vi "MecaDrivePoseEst2_New.vi"(4 "VisionMeasurementStdDevs":T4=[[0.9], [0.9], [0.9]], 6 "StateStdDevs":T4=[[0.1], [0.1], [0.1]], 7 "MECA_DRIVE_KINEMATICS":T2={"FrontLeft"={"X"=0.0, "Y"=0.0}, "FrontRight"={"X"=0.0, "Y"=0.0}, "RearLeft"={"X"=0.0, "Y"=0.0}, "RearRight"={"X"=0.0, "Y"=0.0}, "InverseKinematics"=[[0.0, 1.0, -1.0, 0.0], [0.0, 1.0, 1.0, 0.0], [0.0, 1.0, 1.0, 0.0], [0.0, 1.0, -1.0, 0.0]], "ForwardKinematics"=[[0.0, 1.0, -1.0, 0.0], [0.0, 1.0, 1.0, 0.0], [0.0, 1.0, 1.0, 0.0], [0.0, 1.0, -1.0, 0.0]], "PrevCoR"={"X"=0.0, "Y"=0.0}} {"PrevCoR"."Y" format="%14.3f"; "PrevCoR"."X" format="%14.3f"; "RearRight"."Y" format="%14.3f"; "RearRight"."X" format="%14.3f"; "RearLeft"."Y" format="%14.3f"; "RearLeft"."X" format="%14.3f"; "FrontRight"."Y" format="%14.3f"; "FrontRight"."X" format="%14.3f"; "FrontLeft"."Y" format="%14.3f"; "FrontLeft"."X" format="%14.3f"}, 8 "InitialPose":T5={"TRANSLATION"={"X"=0.0, "Y"=0.0}, "ROTATION"={"VALUE"=0.0, "COS"=1.0, "SIN"=0.0}} {"ROTATION"."SIN" format="%13.4f"; "ROTATION"."COS" format="%13.4f"; "ROTATION"."VALUE" format="%13.4f"; "TRANSLATION"."Y" format="%14.3f"; "TRANSLATION"."X" format="%14.3f"}, 10 "Module Positions":T1 {"RearRight" format="%19.3f"; "RearLeft" format="%19.3f"; "FrontRight" format="%19.3f"; "FrontLeft" format="%19.3f"}, 11 "gyroAngle":T6={"VALUE"=0.0, "COS"=1.0, "SIN"=0.0} {"SIN" format="%13.4f"; "COS" format="%13.4f"; "VALUE" format="%13.4f"}) -> (0 "Error":errorcluster, 3 "MecaDrivePoseEstimate":T7={"M_Vision_K"=[], "m_nominal_dT"=0.0, "m_PrevTime_Sec"=0.0, "Pose_Buffer"={"TimeStamps"=[], "DataArray"=[], "Min_TimeStamp"=0.0, "Max_TimeStamp"=0.0, "ItemCount"=0, "MaxBufferTime"=0.0}, "Meca_Drive_Odom"={"POSE"={"TRANSLATION"={"X"=0.0, "Y"=0.0}, "ROTATION"={"VALUE"=0.0, "COS"=1.0, "SIN"=0.0}}, "GyroOffset"={"VALUE"=0.0, "COS"=1.0, "SIN"=0.0}, "PreviousAngle"={"VALUE"=0.0, "COS"=1.0, "SIN"=0.0}, "Kinematics"={"FrontLeft"={"X"=0.0, "Y"=0.0}, "FrontRight"={"X"=0.0, "Y"=0.0}, "RearLeft"={"X"=0.0, "Y"=0.0}, "RearRight"={"X"=0.0, "Y"=0.0}, "InverseKinematics"=[[0.0, 1.0, -1.0, 0.0], [0.0, 1.0, 1.0, 0.0], [0.0, 1.0, 1.0, 0.0], [0.0, 1.0, -1.0, 0.0]], "ForwardKinematics"=[[0.0, 1.0, -1.0, 0.0], [0.0, 1.0, 1.0, 0.0], [0.0, 1.0, 1.0, 0.0], [0.0, 1.0, -1.0, 0.0]], "PrevCoR"={"X"=0.0, "Y"=0.0}}, "PreviousWheelPositions"={"FrontLeft"=0.0, "FrontRight"=0.0, "RearLeft"=0.0, "RearRight"=0.0, "P"=FALSE}}, "M_Q"=[[0.0], [0.0], [0.0]]} {"Meca_Drive_Odom"."PreviousWheelPositions"."RearRight" format="%19.3f"; "Meca_Drive_Odom"."PreviousWheelPositions"."RearLeft" format="%19.3f"; "Meca_Drive_Odom"."PreviousWheelPositions"."FrontRight" format="%19.3f"; "Meca_Drive_Odom"."PreviousWheelPositions"."FrontLeft" format="%19.3f"; "Meca_Drive_Odom"."Kinematics"."PrevCoR"."Y" format="%14.3f"; "Meca_Drive_Odom"."Kinematics"."PrevCoR"."X" format="%14.3f"; "Meca_Drive_Odom"."Kinematics"."RearRight"."Y" format="%14.3f"; "Meca_Drive_Odom"."Kinematics"."RearRight"."X" format="%14.3f"; "Meca_Drive_Odom"."Kinematics"."RearLeft"."Y" format="%14.3f"; "Meca_Drive_Odom"."Kinematics"."RearLeft"."X" format="%14.3f"; "Meca_Drive_Odom"."Kinematics"."FrontRight"."Y" format="%14.3f"; "Meca_Drive_Odom"."Kinematics"."FrontRight"."X" format="%14.3f"; "Meca_Drive_Odom"."Kinematics"."FrontLeft"."Y" format="%14.3f"; "Meca_Drive_Odom"."Kinematics"."FrontLeft"."X" format="%14.3f"; "Meca_Drive_Odom"."PreviousAngle"."SIN" format="%13.4f"; "Meca_Drive_Odom"."PreviousAngle"."COS" format="%13.4f"; "Meca_Drive_Odom"."PreviousAngle"."VALUE" format="%13.4f"; "Meca_Drive_Odom"."GyroOffset"."SIN" format="%13.4f"; "Meca_Drive_Odom"."GyroOffset"."COS" format="%13.4f"; "Meca_Drive_Odom"."GyroOffset"."VALUE" format="%13.4f"; "Meca_Drive_Odom"."POSE"."ROTATION"."SIN" format="%13.4f"; "Meca_Drive_Odom"."POSE"."ROTATION"."COS" format="%13.4f"; "Meca_Drive_Odom"."POSE"."ROTATION"."VALUE" format="%13.4f"; "Meca_Drive_Odom"."POSE"."TRANSLATION"."Y" format="%14.3f"; "Meca_Drive_Odom"."POSE"."TRANSLATION"."X" format="%14.3f"})   [LabVIEW 2019, in "Trajectory_Library.lvlib"]
doc: "This set of functions wraps MecaDriveOdometry to fuse latency-compensated vision measurements with mecanum drive encoder distance measurements. It will correct for noisy measurements and encoder drift. It is intended to be a drop-in replacement MecaDriveOdometry.\n \nMecaDrivePoseEst2_update should be called every robot loop.\n \nMecaDrivePoseEst2_addVisionMeasurement can be called as infrequently as you want; if you never call it, then this class will behave mostly like regular encoder odometry.\n\nConstructs a MecaDrivePoseEst2.\n\nThe default standard deviations of the model states are 0.1 meters for x, 0.1 meters for y, and 0.1 radians for heading. The default standard deviations of the vision measurements are 0.45 meters for x, 0.45 meters for y, and 0.45 radians for heading.\n\nInputs: \n - kinematics -- MecaDriveKinematics -- A correctly-configured kinematics data cluster for your drivetrain.\n - gyroAngle -- Rotation2d -- The current gyro angle.\n - ModulePositions -- ModulePositions -- The current module positions.\n - initialPoseMeters -- Pose2d -- The starting pose estimate.\n - stateStdDevs -- <3,1> matrix -- Standard deviations of the pose estimate (x position in meters, y position in meters, and heading in radians). Increase these numbers to trust your state estimate less.\n - visionMeasurementStdDevs -- <3,1> matrix -- Standard deviations of the vision pose measurement (x position in meters, y position in meters, and heading in radians). Increase these numbers to trust the vision pose measurement less.\n \nOutputs:\n -- MecaDrivePoseEst2 -- MecaDrivePoseEst2 -- Created data cluster."
uses:
  Trajectory_Library.lvlib
  TypeDef/MECA_DRIVE_POSE_EST2.ctl
  <vilib>/Analysis/Matrix/Datatypes/RealMatrix.ctl
  TypeDef/TIME_INTERPOLATABLE_VARIANT.ctl
  TypeDef/MECA_DRIVE_ODOMETRY.ctl
  TypeDef/POSE2D.ctl
  TypeDef/TRANSLATION2D.ctl
  TypeDef/ROTATION2D.ctl
  TypeDef/MECA_DRIVE_KINEMATICS.ctl
  TypeDef/MECA_WHEEL_POSITIONS.ctl
  MatBuilder_Create.vi
  Matrix_Create.vi
  <vilib>/Analysis/Matrix/NI_Matrix.lvlib
panel:
  # "<3,1>"
  # "<3, 1>"
  # "<3, 1>"
  # "<3, 3>"
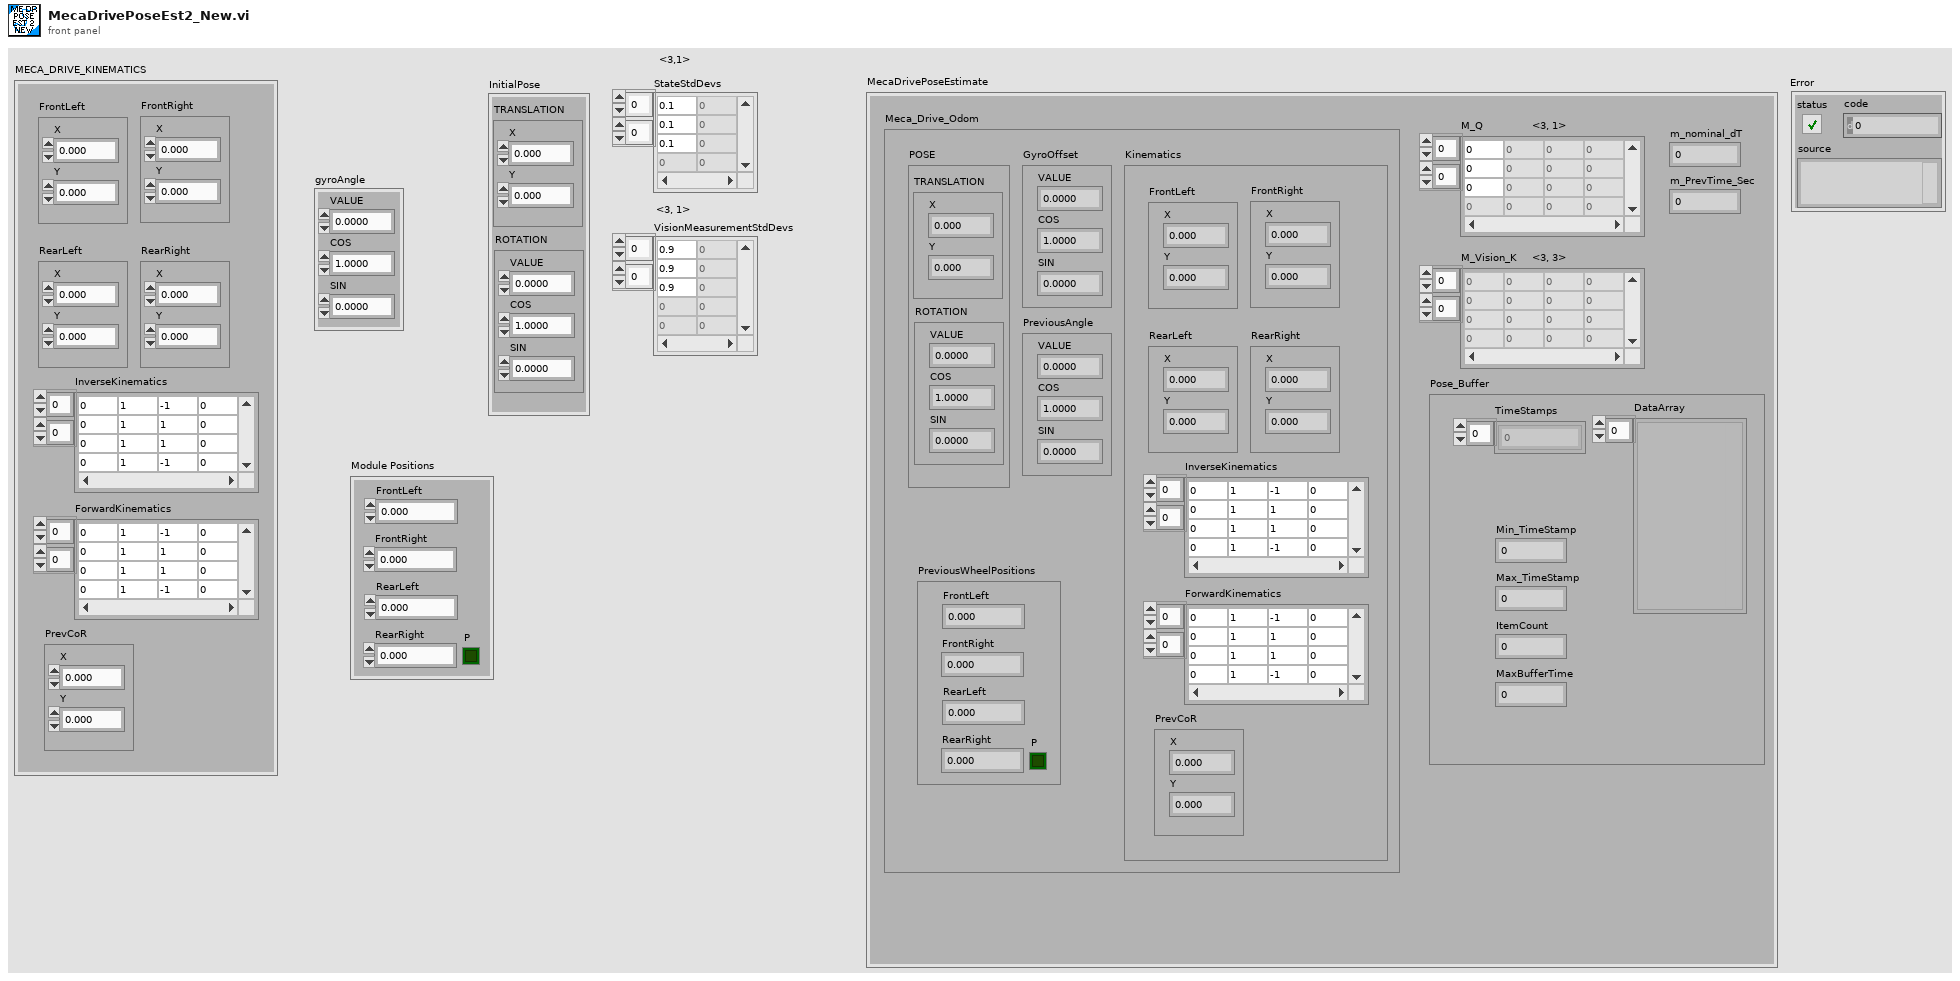
[diagram p1: front panel]
types:
  T1 = typedef "Trajectory_Library.lvlib/MECA_WHEEL_POSITIONS.ctl" = cluster{"FrontLeft":dbl, "FrontRight":dbl, "RearLeft":dbl, "RearRight":dbl, "P":bool}
  T2 = typedef "Trajectory_Library.lvlib/MECA_DRIVE_KINEMATICS.ctl" = cluster{"FrontLeft":T3, "FrontRight":T3, "RearLeft":T3, "RearRight":T3, "InverseKinematics":T4, "ForwardKinematics":T4, "PrevCoR":T3}
  T3 = typedef "Trajectory_Library.lvlib/TRANSLATION2D.ctl" = cluster{"X":dbl, "Y":dbl}
  T4 = typedef "NI_Matrix.lvlib/RealMatrix.ctl" = dbl[][]
  T5 = typedef "Trajectory_Library.lvlib/POSE2D.ctl" = cluster{"TRANSLATION":T3, "ROTATION":T6}
  T6 = typedef "Trajectory_Library.lvlib/ROTATION2D.ctl" = cluster{"VALUE":dbl, "COS":dbl, "SIN":dbl}
  T7 = typedef "Trajectory_Library.lvlib/MECA_DRIVE_POSE_EST2.ctl" = cluster{"M_Vision_K":T4, "m_nominal_dT":dbl, "m_PrevTime_Sec":dbl, "Pose_Buffer":T8, "Meca_Drive_Odom":T9, "M_Q":T4}
  T8 = typedef "Trajectory_Library.lvlib/TIME_INTERPOLATABLE_VARIANT.ctl" = cluster{"TimeStamps":dbl[], "DataArray":variant[], "Min_TimeStamp":dbl, "Max_TimeStamp":dbl, "ItemCount":i32, "MaxBufferTime":dbl}
  T9 = typedef "Trajectory_Library.lvlib/MECA_DRIVE_ODOMETRY.ctl" = cluster{"POSE":T5, "GyroOffset":T6, "PreviousAngle":T6, "Kinematics":T2, "PreviousWheelPositions":T1}
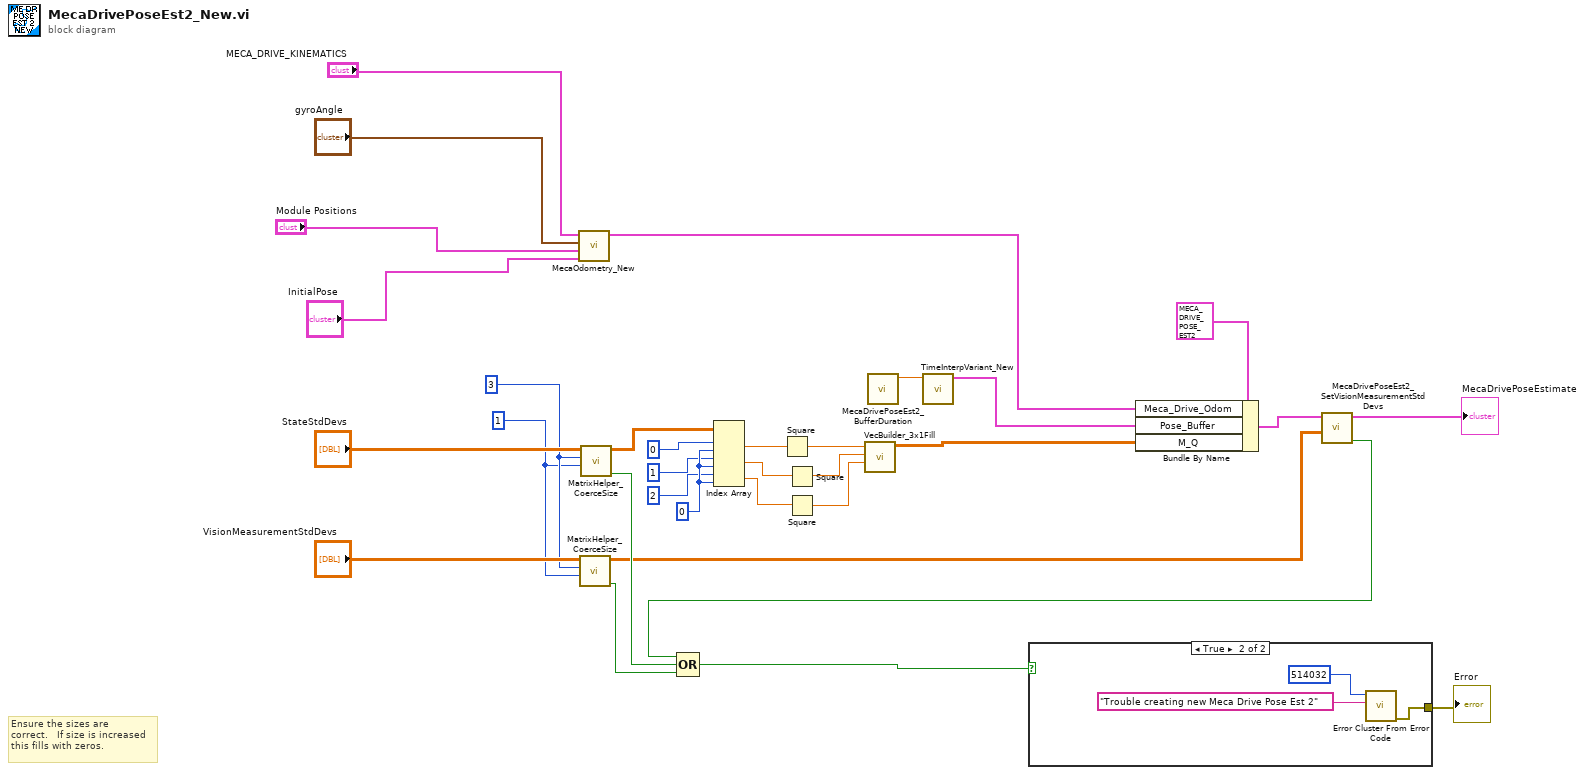
[diagram p0: block diagram]
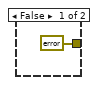
[diagram p2: hidden frame]
diagram:
  w19 = 0 ("index (col)")
  w22 = 1 ("Outputs")
  w23 = 3 ("States")
  # "Ensure the sizes are\ncorrect.   If size is increased \nthis fills with zeros."
  n1 = call "MecaOdometry_New.vi"("Initial Pose2d"="InitialPose", "wheelPositions"="Module Positions", "GyroOffset"="gyroAngle", "Mecanum Kinematics"="MECA_DRIVE_KINEMATICS") -> ("MECA_DRIVE_ODOMETRY"=w25:T9)  [unwired: 7 in]
  n2 = call "MatrixHelper_CoerceSize.vi"("Columns"=w22, "Rows"=w23, "input matrix"="VisionMeasurementStdDevs") -> ("Coerced"=w9:bool, "output matrix"=w6:T4)  [unwired: 7 in]
  n3 = call "MatrixHelper_CoerceSize.vi"("Columns"=w22, "Rows"=w23, "input matrix"="StateStdDevs") -> ("Coerced"=w30:bool, "output matrix"=w21:T4)  [unwired: 7 in]
  n4 = Index Array(array=w21, index (row) #1=0 ("index (row)"), index (col) #1=w19, index (row) #2=1 ("index (row)"), index (col) #2=w19, index (row) #3=2 ("index (row)"), index (col) #3=w19) -> (element #1=w16:dbl, element #2=w15:dbl, element #3=w14:dbl)
  n5 = Square(x=w16) -> (x^2=w13:dbl)
  n6 = Square(x=w15) -> (x^2=w12:dbl)
  n7 = Square(x=w14) -> (x^2=w11:dbl)
  n8 = call "VecBuilder_3x1Fill.vi"("R2"=w11, "R1"=w12, "R0"=w13) -> ("output matrix"=w10:T4)  [unwired: 8 in]
  n9 = call "MecaDrivePoseEst2_BufferDuration.vi"() -> ("Buffer Duration (Sec)"=w5:dbl)  [unwired: 11 in]
  n10 = call "TimeInterpVariant_New.vi"("MaxTime"=w5) -> ("TimeInterpVariant"=w24:T8)  [unwired: 10 in]
  n11 = Bundle By Name(cluster=T7 {"M_Vision_K"=[], "m_nominal_dT"=0.0, "m_PrevTime_Sec"=0.0, "Pose_Buffer"={"TimeStamps"=[], "DataArray"=[], "Min_TimeStamp"=0.0, "Max_TimeStamp"=0.0, "ItemCount"=0, "MaxBufferTime"=0.0}, "Meca_Drive_Odom"={"POSE"={"TRANSLATION"={"X"=0.0, "Y"=0.0}, "ROTATION"={"VALUE"=0.0, "COS"=1.0, "SIN"=0.0}}, "GyroOffset"={"VALUE"=0.0, "COS"=1.0, "SIN"=0.0}, "PreviousAngle"={"VALUE"=0.0, "COS"=1.0, "SIN"=0.0}, "Kinematics"={"FrontLeft"={"X"=0.0, "Y"=0.0}, "FrontRight"={"X"=0.0, "Y"=0.0}, "RearLeft"={"X"=0.0, "Y"=0.0}, "RearRight"={"X"=0.0, "Y"=0.0}, "InverseKinematics"=[[0.0, 1.0, -1.0, 0.0], [0.0, 1.0, 1.0, 0.0], [0.0, 1.0, 1.0, 0.0], [0.0, 1.0, -1.0, 0.0]], "ForwardKinematics"=[[0.0, 1.0, -1.0, 0.0], [0.0, 1.0, 1.0, 0.0], [0.0, 1.0, 1.0, 0.0], [0.0, 1.0, -1.0, 0.0]], "PrevCoR"={"X"=0.0, "Y"=0.0}}, "PreviousWheelPositions"={"FrontLeft"=0.0, "FrontRight"=0.0, "RearLeft"=0.0, "RearRight"=0.0, "P"=FALSE}}, "M_Q"=[[0.0], [0.0], [0.0]]} ("DiffDrivePoseEstimate 2"), "Meca_Drive_Odom"=w25, "Pose_Buffer"=w24, "M_Q"=w10) -> (w4:T7)
  n12 = call "MecaDrivePoseEst2_SetVisionMeasurementStdDevs.vi"("VisionMeasurementStdDevs"=w6, "in MecaDrivePoseEstimate2"=w4) -> ("Size Coerced"=w7:bool, "Out MecaDrivePoseEstimate2"=→"MecaDrivePoseEstimate":T7)  [unwired: 8 in]
  n13 = Compound Arithmetic op=OR(w7, w30, w9) -> (w8:bool)
  n14 = case shown="True" w8 {
    tunnel: [errorcluster {"status"=FALSE, "code"=0, "source"=""} ("error out") w36] -> w29
    frame False {
    }
    frame True {
      n15 = call <vilib>:"Error Cluster From Error Code.vi"("error message (\"\")"="Trouble creating new Meca Drive Pose Est 2" ("error message (\"\")"), "error code (0)"=514032) -> ("error out"=w36:errorcluster)  [unwired: 7 in]
    }
  }
  "Error" <- w29
